vi "Resolve Inset ID.vi"(8 "error in":errorcluster, 11 "Inset in":refnum<class "Inset.lvclass">) -> (0 "error out":errorcluster, 3 "Inset out":refnum<class "Inset.lvclass">)   [LabVIEW 2019, in "Inset.lvclass"]
uses:
  Inset.lvclass
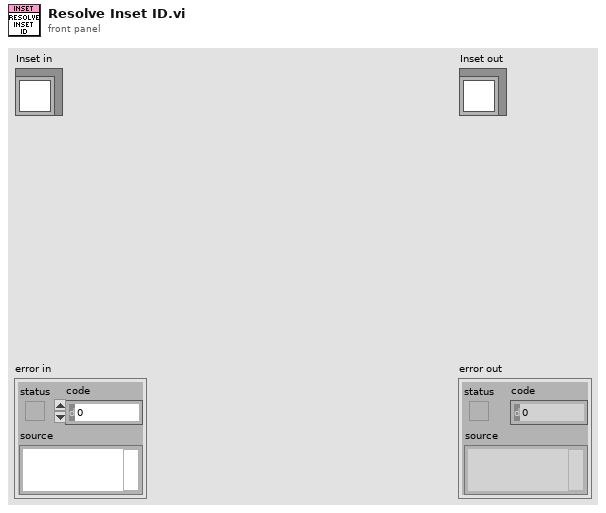
[diagram p1: front panel]
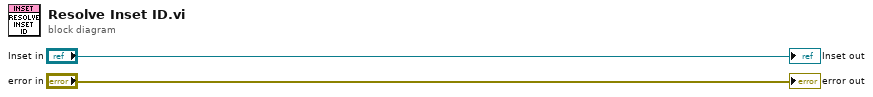
[diagram p0: block diagram]
diagram:
  "error out" <- "error in"
  "Inset out" <- "Inset in"
